vi "Pointer-to-C-String to String.vi"(8 "error in (no error)":errorcluster, 10 "Max Length":i32, 11 "Pointer to C-String":u64) -> (0 "error out":errorcluster, 3 "String":string)   [LabVIEW 2023, in "SQLite.lvlib"]
doc: "Uses the MemCopy funtion of LabVIEW.exe to copy data from a pointer location, then truncate it at the first zero byte (indicating the end of a C-formate string). Returns the resut as a standard LabVIEW String."
uses:
  SQLite.lvlib
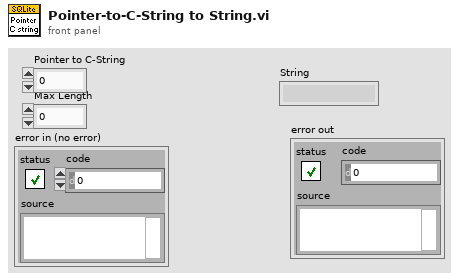
[diagram p1: front panel]
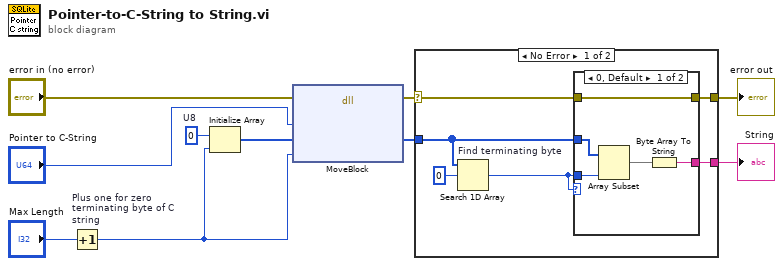
[diagram p0: block diagram]
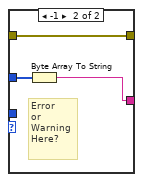
[diagram p2: hidden frame]
diagram:
  w9 = u8 0  # U8
  n1 = Increment "Plus one for zero terminating byte of C string"(x="Max Length") -> (x+1=w6:i32)
  n2 = Initialize Array "Initialize Array"(w9, w6) -> (w10:u8[])
  n3 = dll-call lib="LabVIEW" fn="MoveBlock"(error in="error in (no error)", "Source Pointer"="Pointer to C-String", "Destination U8 Array"=w10, "Number of Bytes"=w6) -> (error out=w2:errorcluster, "Destination U8 Array"=w8:u8[])  [unwired: 5 in, 1 out]
  n4 = case shown="No Error" w2 {
    selector: w2 -> [w12 w25]
    tunnel: w8 -> [w15 _]
    tunnel: [w14 _] -> w4
    tunnel: [w11 w25] -> w1
    frame No Error {
      n5 = Search 1D Array "Find terminating byte"(1D array=w15, element=u8 0) -> (index of element=w13:i32)  [unwired: 1 in]
      n6 = case shown="0, Default" w13 {
        tunnel: w15 -> [w21 w24]
        tunnel: w13 -> [w19 _]
        tunnel: [w18 w23] -> w14
        tunnel: w12 -> [w17 w22]
        tunnel: [w17 w22] -> w11
        frame 0, Default {
          n7 = Array Subset(array=w21, length=w19) -> (w20:u8[])  [unwired: 1 in]
          n8 = Byte Array To String(unsigned byte array=w20) -> (string=w18:string)
        }
        frame -1 {
          # "Error\nor\nWarning\nHere?"
          n9 = Byte Array To String(unsigned byte array=w24) -> (string=w23:string)
        }
      }
    }
    frame Error {
    }
  }
  "String" <- w4
  "error out" <- w1
